vi "WPI_CounterOpen & Configure.vi"(4 "External Reset Active High":bool=TRUE, 6 "External Reset":T1={"DevStatus"={"status"=FALSE, "code"=0, "source"=""}, "AnalogTriggerMode?"=FALSE, "DigitalMode"={"DIO Channel"=enum."Disabled"}, "AnalogTriggerMode"={"AnalogTriggerIndex"=enum."Trig 0", "OutputType"=enum."InWindow"}}, 7 "GTSDirThreshold":sgl=5.5e-05, 8 "error in (no error)":errorcluster, 9 "EdgeType":T5={"Master Mode"=enum."Edge Detection", "UpChannel"=enum."Disabled", "DownChannel"=enum."Disabled", "High/Up"=FALSE}, 10 "Down Source":T1={"DevStatus"={"status"=FALSE, "code"=0, "source"=""}, "AnalogTriggerMode?"=FALSE, "DigitalMode"={"DIO Channel"=enum."Disabled"}, "AnalogTriggerMode"={"AnalogTriggerIndex"=enum."Trig 0", "OutputType"=enum."InWindow"}}, 11 "Up Source":T1={"DevStatus"={"status"=FALSE, "code"=0, "source"=""}, "AnalogTriggerMode?"=FALSE, "DigitalMode"={"DIO Channel"=enum."Disabled"}, "AnalogTriggerMode"={"AnalogTriggerIndex"=enum."Trig 0", "OutputType"=enum."InWindow"}}) -> (0 "error out":errorcluster, 3 "CounterDevRef":T6)   [LabVIEW 2017]
doc: "This software is licensed. Open the labview\\readme\\WPI Robotics Library Open Source License.txt file for more information."
uses:
  <vilib>/Rock Robotics/WPI/Counter/WPI_CounterDevRef.ctl
  <vilib>/Rock Robotics/SystemInterfaces/Counter/FPGA_CounterCtrSystemIndex.ctl
  <vilib>/Rock Robotics/SystemInterfaces/Counter/FPGA_CounterCtrEdgeDetectionType.ctl
  <vilib>/Rock Robotics/SystemInterfaces/CounterEncoderSourceConvertion/FPGA_CounterEncoderSourceConvertionLVSourceType.ctl
  <vilib>/Rock Robotics/SystemInterfaces/DIO/FPGA_DIODigitalSourceChannel.ctl
  <vilib>/Rock Robotics/SystemInterfaces/AnalogTrigger/FPGA_AnalogTriggerIndex.ctl
  <vilib>/Rock Robotics/SystemInterfaces/AnalogTrigger/FPGA_AnalogTriggerOutType.ctl
  <vilib>/Rock Robotics/WPI/Counter/WPI_CounterCacheOp.ctl
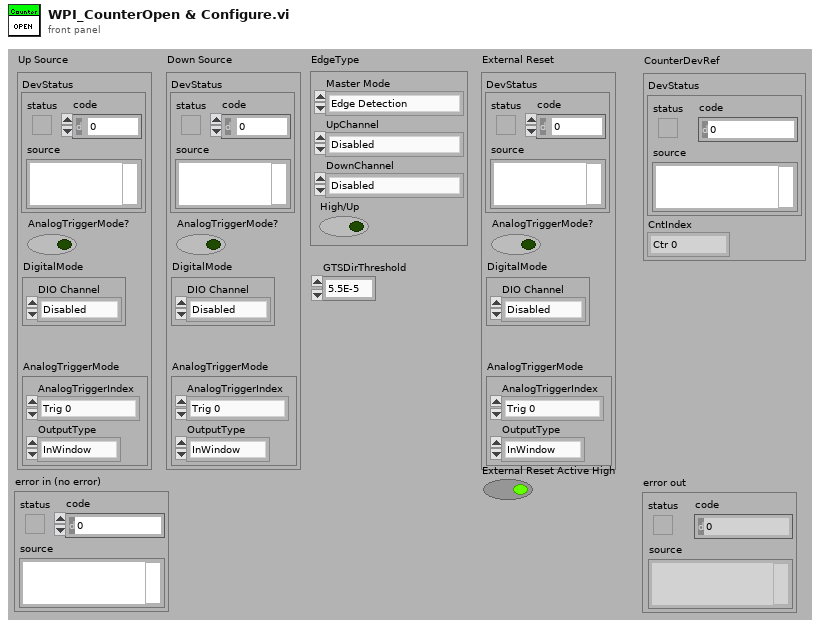
[diagram p1: front panel]
types:
  T1 = typedef "FPGA_CounterEncoderSourceConvertionLVSourceType.ctl" = cluster{"DevStatus":errorcluster, "AnalogTriggerMode?":bool, "DigitalMode":cluster{"DIO Channel":T2}, "AnalogTriggerMode":cluster{"AnalogTriggerIndex":T3, "OutputType":T4}}
  T2 = typedef "FPGA_DIODigitalSourceChannel.ctl" = enum8{"DIO 0", "DIO 1", "DIO 2", "DIO 3", "DIO 4", "DIO 5", "DIO 6", "DIO 7", "DIO 8", "DIO 9", "DIO MXP 0", "DIO MXP 1", "DIO MXP 2", "DIO MXP 3", "DIO MXP 4", "DIO MXP 5", "DIO MXP 6", "DIO MXP 7", "DIO MXP 8", "DIO MXP 9", "DIO MXP 10", "DIO MXP 11", "DIO MXP 12", "DIO MXP 13", "DIO MXP 14", "DIO MXP 15", "Disabled"}
  T3 = typedef "FPGA_AnalogTriggerIndex.ctl" = enum8{"Trig 0", "Trig 1", "Trig 2", "Trig 3", "Trig 4", "Trig 5", "Trig 6", "Trig 7", "Invalid"}
  T4 = typedef "FPGA_AnalogTriggerOutType.ctl" = enum16{"InWindow", "TriggerState", "Rising", "Falling"}
  T5 = typedef "FPGA_CounterCtrEdgeDetectionType.ctl" = cluster{"Master Mode":enum16{"Edge Detection", "Semi Period Mode", "Pulse Length Mode", "External Direction"}, "UpChannel":enum16{"Rising Edge", "Falling Edge", "Raising & Falling Edge", "Disabled"}, "DownChannel":enum16{"Rising Edge", "Falling Edge", "Raising & Falling Edge", "Disabled"}, "High/Up":bool}
  T6 = typedef "WPI_CounterDevRef.ctl" = cluster{"DevStatus":errorcluster, "CntIndex":T7}
  T7 = typedef "FPGA_CounterCtrSystemIndex.ctl" = enum8{"Ctr 0", "Ctr 1", "Ctr 2", "Ctr 3", "Ctr 4", "Ctr 5", "Ctr 6", "Ctr 7", "Invalid"}
  T8 = typedef "WPI_CounterCacheOp.ctl" = enum16{"Acquire", "Release"}
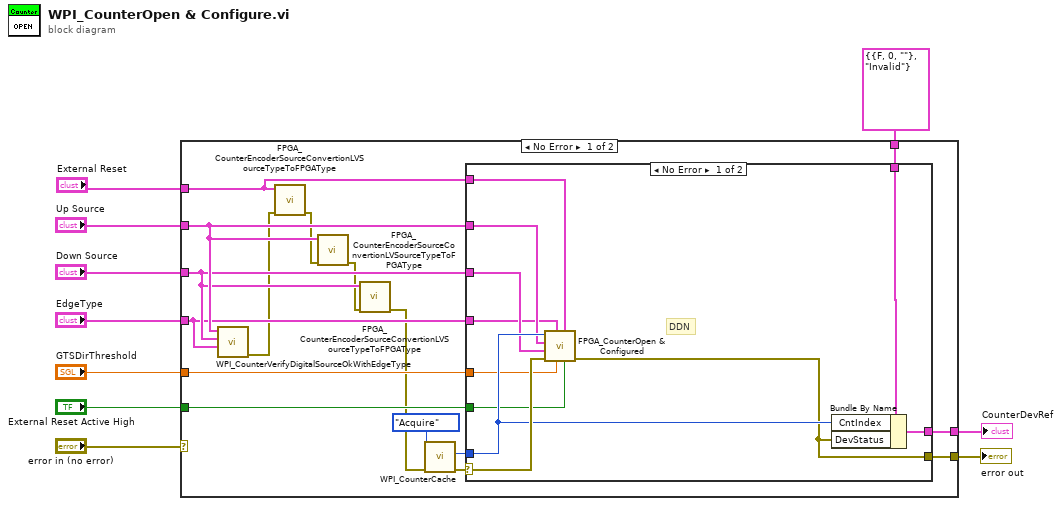
[diagram p0: block diagram]
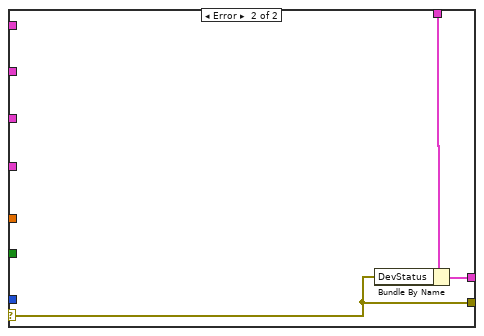
[diagram p2: hidden frame]
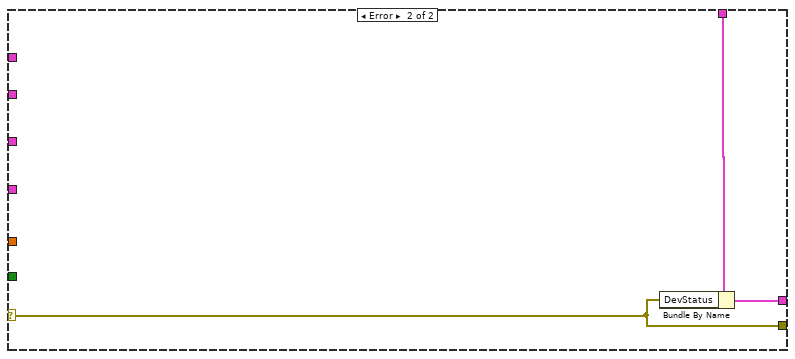
[diagram p3: hidden frame]
diagram:
  n1 = case shown="No Error" "error in (no error)" {
    selector: "error in (no error)" -> [_ w41]
    tunnel: [w26 w42] -> w10
    tunnel: T6 {"DevStatus"={"status"=FALSE, "code"=0, "source"=""}, "CntIndex"=enum."Invalid"} ("CounterDevRef") -> [w25 w43]
    tunnel: [w24 w41] -> w7
    tunnel: "EdgeType" -> [w15 _]
    tunnel: "Up Source" -> [w17 _]
    tunnel: "Down Source" -> [w16 _]
    tunnel: "GTSDirThreshold" -> [w20 _]
    tunnel: "External Reset" -> [w19 _]
    tunnel: "External Reset Active High" -> [w18 _]
    frame No Error {
      n2 = call <vilib>:"WPI_CounterVerifyDigitalSourceOkWithEdgeType.vi"("EdgeType"=w15, "Down Source"=w16, "Up Source"=w17) -> ("error out"=w12:errorcluster)  [unwired: 8 out]
      n3 = call <vilib>:"FPGA_CounterEncoderSourceConvertionLVSourceTypeToFPGAType.vi"("error in (no error)"=w12, "DigitalSource"=w19) -> ("error out"=w14:errorcluster)  [unwired: 9 out]
      n4 = call <vilib>:"FPGA_CounterEncoderSourceConvertionLVSourceTypeToFPGAType.vi"("error in (no error)"=w14, "DigitalSource"=w17) -> ("error out"=w13:errorcluster)  [unwired: 9 out]
      n5 = call <vilib>:"FPGA_CounterEncoderSourceConvertionLVSourceTypeToFPGAType.vi"("error in (no error)"=w13, "DigitalSource"=w16) -> ("error out"=w11:errorcluster)  [unwired: 9 out]
      n6 = call <vilib>:"WPI_CounterCache.vi"("error in (no error)"=w11, "Operation"=WPI_CounterCacheOp."Acquire") -> ("error out"=w22:errorcluster, "CntIndexAllocated"=w21:T7)  [unwired: 1 in, 7 out]
      n7 = case shown="No Error" w22 {
        selector: w22 -> [w35 w38]
        tunnel: [w37 w39] -> w26
        tunnel: w25 -> [w36 w40]
        tunnel: [w27 w38] -> w24
        tunnel: w21 -> [w34 _]
        tunnel: w15 -> [w28 _]
        tunnel: w17 -> [w33 _]
        tunnel: w16 -> [w32 _]
        tunnel: w20 -> [w31 _]
        tunnel: w19 -> [w30 _]
        tunnel: w18 -> [w29 _]
        frame No Error {
          # "DDN"
          n8 = call <vilib>:"FPGA_CounterOpen & Configured.vi"("IndexActiveHigh"=w29, "External Reset"=w30, "GTSDirThreshold"=w31, "EdgeType"=w28, "error in"=w35, "DownSource"=w32, "UpSource"=w33, "CntIndex"=w34) -> ("error out"=w27:errorcluster)  [unwired: 1 in, 2 out]
          n9 = Bundle By Name(cluster=w36, "CntIndex"=w34, "DevStatus"=w27) -> (w37:T6)
        }
        frame Error {
          n10 = Bundle By Name(cluster=w40, "DevStatus"=w38) -> (w39:T6)
        }
      }
    }
    frame Error {
      n11 = Bundle By Name(cluster=w43, "DevStatus"=w41) -> (w42:T6)
    }
  }
  "CounterDevRef" <- w10
  "error out" <- w7
